vi "Draw+.vi"(1 "Width":i32=25, 2 "Color":u32(colorbox)=16711680, 3 "Pos_Y":i32, 4 "Pos_X":i32, 5 "input cluster":cluster{"P_X":i32, "P_Y":i32}, 6 "Image In":T1) -> (0 "Image Out":T1)   [LabVIEW 2014]
uses:
  <vilib>/vision/Image Controls.llb/IMAQ Image.ctl
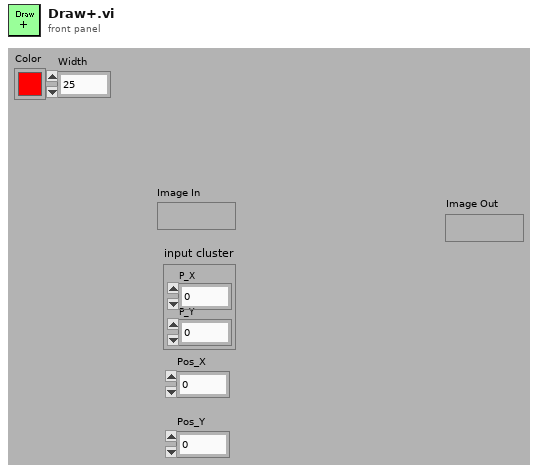
[diagram p1: front panel]
types:
  T1 = typedef "IMAQ Image.ctl" = refnum<image>
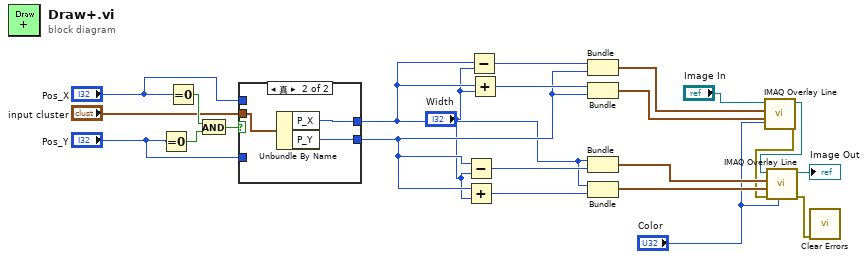
[diagram p0: block diagram]
diagram:
  n1 = Equal To 0?(x="Pos_Y") -> (x = 0?=w22:bool)
  n2 = Equal To 0?(x="Pos_X") -> (x = 0?=w23:bool)
  n3 = And(x=w23, y=w22) -> (x .and. y?=w21:bool)
  n4 = case shown="真" w21 {
    tunnel: "input cluster" -> [_ w28]
    tunnel: [w25 w27] -> w9
    tunnel: [w24 w26] -> w13
    tunnel: "Pos_X" -> [w25 _]
    tunnel: "Pos_Y" -> [w24 _]
    frame False {
    }
    frame True {
      n5 = Unbundle By Name(w28) -> ("P_X"=w27:i32, "P_Y"=w26:i32)
    }
  }
  n6 = Subtract(x=w13, y="Width") -> (x-y=w11:i32)
  n7 = Add(x=w13, y="Width") -> (x+y=w10:i32)
  n8 = Subtract(x=w9, y="Width") -> (x-y=w17:i32)
  n9 = Add(x=w9, y="Width") -> (x+y=w14:i32)
  n10 = Bundle(w17, "P_Y"=w13) -> (w15:cluster{i32, "P_Y":i32})  [unwired: 1 in]
  n11 = Bundle(w14, "P_Y"=w13) -> (w12:cluster{i32, "P_Y":i32})  [unwired: 1 in]
  n12 = Bundle("P_X"=w9, w11) -> (w7:cluster{"P_X":i32, i32})  [unwired: 1 in]
  n13 = Bundle("P_X"=w9, w10) -> (w6:cluster{"P_X":i32, i32})  [unwired: 1 in]
  n14 = call "IMAQ Overlay Line"("Color"="Color", "End Point"=w12, "Start Point"=w15, "Image"="Image In") -> ("error out"=w1:errorcluster, "Image Out"=w8:T1)  [unwired: 6 in]
  n15 = call "IMAQ Overlay Line"("Color"="Color", "error in (no error)"=w1, "End Point"=w6, "Start Point"=w7, "Image"=w8) -> ("error out"=w2:errorcluster, "Image Out"=→"Image Out":T1)  [unwired: 5 in]
  n16 = call <vilib>:"Clear Errors.vi"("error in (no error)"=w2) -> ()  [unwired: 5 in, 2 out]
